vi "YAFTAF_GetExternalInterfaces.vi"(8 "ErrorIn":errorcluster, 10 "CmdData":variant, 11 "LocalIn":refnum<class>) -> (0 "ErrorOut":errorcluster, 2 "ReplyData":variant, 3 "LocalIn":refnum<class>, 4 "Exit":bool)   [LabVIEW 2021, in "YAFTAF.lvclass"]
uses:
  YAFTAF.lvclass
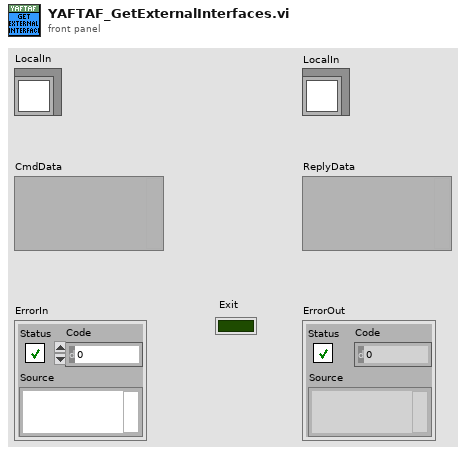
[diagram p1: front panel]
types:
  T1 = typedef "ClusterArrayConversion.lvlib/BundledArray.ctl" = cluster{"Label":string, "Object":refnum<class>, "Array":bool}
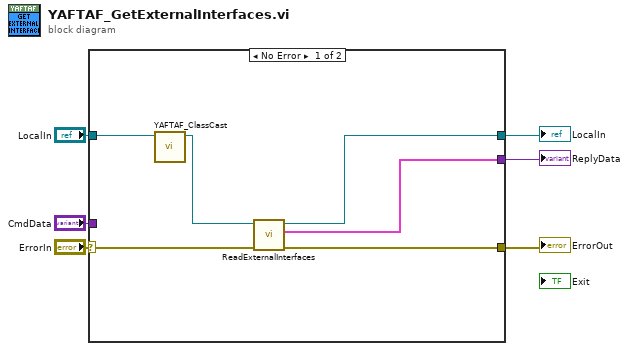
[diagram p0: block diagram]
diagram:
  n1 = case shown="No Error" "ErrorIn" {
    selector: "ErrorIn" -> [w12 w15]
    tunnel: [w11 w15] -> w5
    tunnel: [w7 w14] -> w3
    tunnel: "CmdData" -> [_ w14]
    tunnel: "LocalIn" -> [w10 w13]
    tunnel: [w8 w13] -> w1
    frame No Error {
      n2 = call "YAFTAF_ClassCast.vi"("LocalIn"=w10) -> ("LocalOut"=w9:refnum<class "YAFTAF.lvclass">)  [unwired: 10 in]
      n3 = call-dynamic "ReadExternalInterfaces.vi"("ErrorIn"=w12, "ObjectIn"=w9) -> ("ErrorOut"=w11:errorcluster, "ExternalInterfaces"=w7:T1[], "ObjectOut"=w8:refnum<class "YAFTAF.lvclass">)  [unwired: 7 in]
    }
    frame Error {
    }
  }
  "ErrorOut" <- w5
  "LocalIn" <- w1
  "ReplyData" <- w3
